vi "Open_Instr.vi"(8 "error in (no error)":errorcluster caption="entrée d'erreur (pas d'erreur)", 11 "Class Multimeter Multimeter en entrée":refnum<class "Class Instrument Multimeter.lvclass">) -> (0 "error out":errorcluster caption="sortie d'erreur", 3 "Class Multimeter Multimeter en sortie":refnum<class "Class Instrument Multimeter.lvclass">)   [LabVIEW 2020, in "Library Instrument & Equipement.lvlib" / "Library Instruments.lvlib" / "Class Instrument Multimeter.lvclass"]
uses:
  Class Instrument Multimeter.lvclass
  Class Instrument Multimeter.lvclass/Class Instrument Multimeter.ctl
  Instrument (Default)/Class Instrument (Default).lvclass
  Multimeter/Multimeter (Default)/Class Multimeter (Default).lvclass
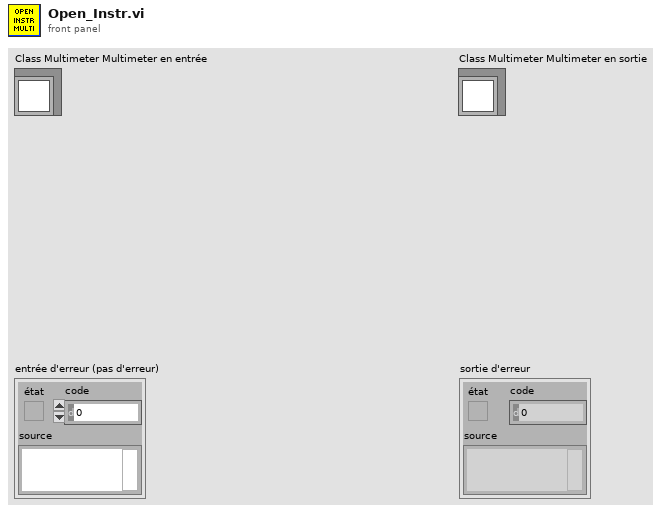
[diagram p1: front panel]
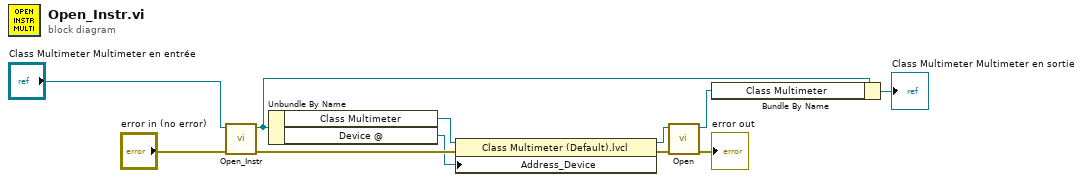
[diagram p0: block diagram]
diagram:
  n1 = call-parent "Open_Instr.vi"("error in (no error)"="error in (no error)", "Class Multimeter (Default) en entrée"="Class Multimeter Multimeter en entrée") -> ("error out"=w7:errorcluster, "Class Multimeter (Default) en sortie"=w3:refnum<class "Class Instrument Multimeter.lvclass">)  [unwired: 8 in]
  n2 = Unbundle By Name(w3) -> ("Class Multimeter"=w8:refnum<class "Class Multimeter (Default).lvclass">, "Device @"=w5:refnum<visa-resource-name>)
  n3 = property class="Class Multimeter (Default).lvcl"(reference=w8, error in=w7, "Address_Device"=w5) -> (reference out=w2:refnum<class "Class Multimeter (Default).lvclass">, error out=w6:errorcluster)
  n4 = call-dynamic "Open.vi"("error in (no error)"=w6, "Class Multimeter (Default) en entrée"=w2) -> ("error out"=→"error out":errorcluster, "Class Multimeter (Default) en sortie"=w1:refnum<class "Class Multimeter (Default).lvclass">)  [unwired: 8 in]
  n5 = Bundle By Name(cluster=w3, "Class Multimeter"=w1) -> (→"Class Multimeter Multimeter en sortie":refnum<class "Class Instrument Multimeter.lvclass">)
